vi "GetIndirectDeps.vi"(8 "error in (no error)":errorcluster, 9 "String":string, 10 "Descendents SubVIs Qualified Name":string[][](array[string]), 11 "LV Descendents Qualified Name":string[](array[string])) -> (0 "error out":errorcluster, 1 "Dependency Chain [] 2":string[](array[string]))   [LabVIEW 2019, in "Hawkeye.lvlib"]
uses:
  e77ed756-b53e-49ae-a6b8-d87d114e66a3.vi
  Hawkeye.lvlib
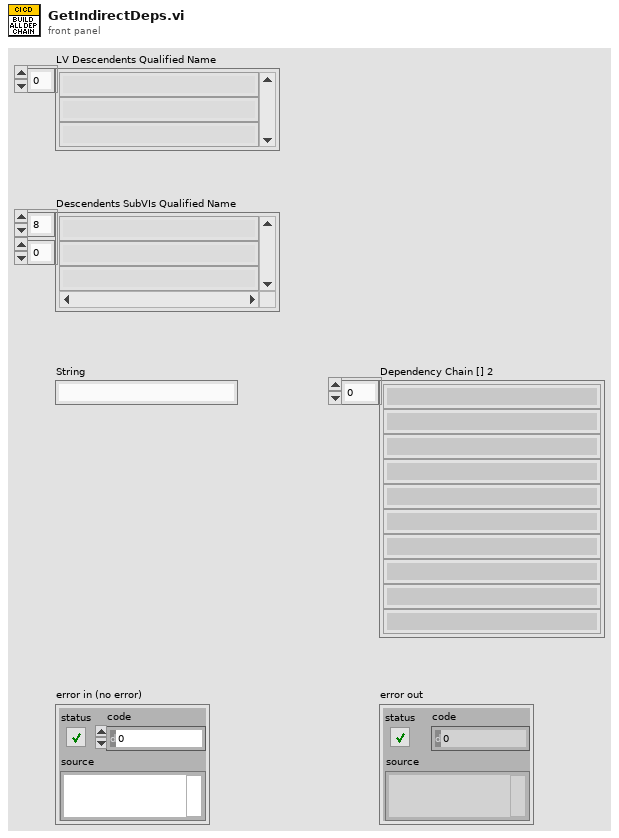
[diagram p1: front panel]
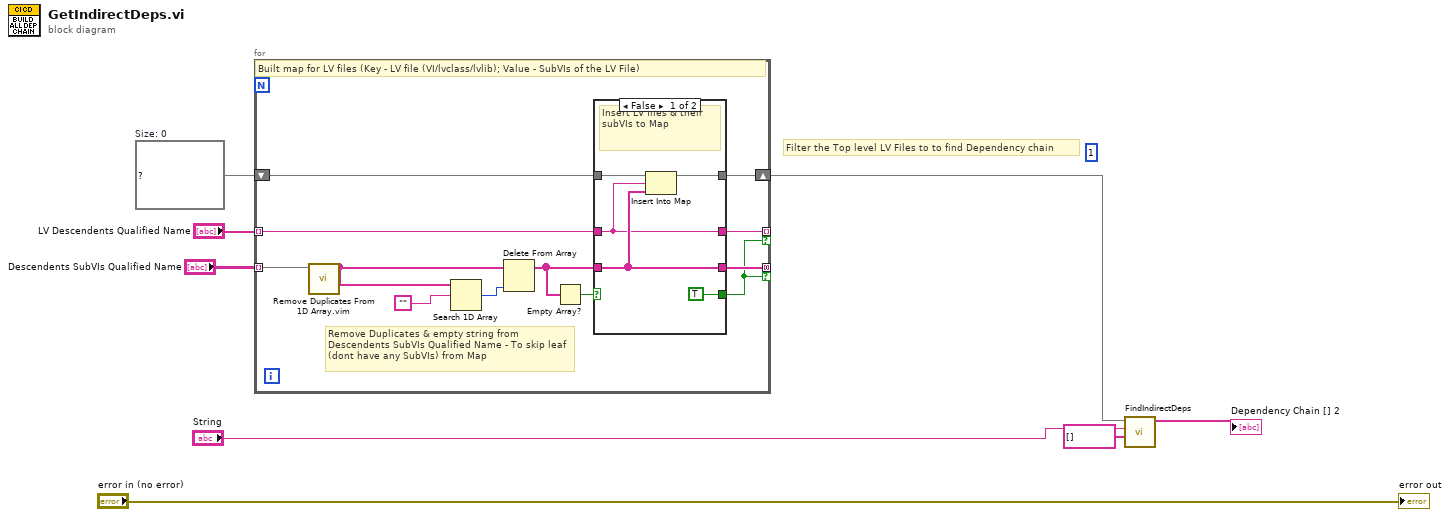
[diagram p0: block diagram]
diagram:
  (unwired) 1
  w8 = map{string, string[]} {}  # Size: 0
  # "Filter the Top level LV Files to to find Dependency chain"
  n1 = for {
    tunnel: "Descendents SubVIs Qualified Name" -> [w9] mode=indexing
    tunnel: "LV Descendents Qualified Name" -> [w14] mode=indexing
    shift-right: [w20] -> w4
    shift-left: w8 -> [w19]
    tunnel: [w12] -> _ mode=concatenating if=w10
    tunnel: [w11] -> _ mode=indexing if=w10
    # "Remove Duplicates & empty string from \nDescendents SubVIs Qualified Name - To skip leaf (dont have any SubVIs) from Map"
    # "Built map for LV files (Key - LV file (VI/lvclass/lvlib); Value - SubVIs of the LV File)"
    n2 = call "Remove Duplicates From 1D Array.vim"("array"=w9) -> ("array with duplicates removed"=w16:string[])  [unwired: 10 in]
    n3 = Search 1D Array(1D array=w16, element="") -> (index of element=w17:i32)  [unwired: 1 in]
    n4 = Delete From Array(array=w16, index=w17) -> (array with subset deleted=w13:string[])  [unwired: 1 in, 1 out]
    n5 = Empty Array?(array=w13) -> (empty?=w15:bool)
    n6 = case shown="False" w15 {
      tunnel: [w25 w26] -> w20
      tunnel: w19 -> [w24 w26]
      tunnel: w14 -> [w22 _]
      tunnel: w13 -> [w23 _]
      tunnel: [w23 _] -> w12
      tunnel: [w22 _] -> w11
      tunnel: [TRUE _] -> w10
      frame False {
        # "Insert LV files & their subVIs to Map"
        n7 = Insert Into Map(map in=w24, key=w22, value=w23) -> (map out=w25:map{string, string[]})  [unwired: 2 out]
      }
      frame True {
      }
    }
  }
  n8 = call "FindIndirectDeps.vi"("Dependency"=string[] [], "Current Dependency"="String", "Dependency Map"=w4) -> ("Dependency Chain []"=→"Dependency Chain [] 2":string[])  [unwired: 8 in]
  "error out" <- "error in (no error)"
